vi "USBData_initialize.vi"(0 "USBData in":refnum<class "USBData.lvclass">, 2 "SeriesSetting":T2(array[cluster]) {"terminal type" items=["Default"=-1, "RSE"=10083, "NRSE"=10078, "Differential"=10106, "Pseudodifferential"=12529]}, 5 "BasePath":path, 7 "RunName":string, 9 "FileName":string, 11 "error in (no error)":errorcluster, 12 "RUN start time":timestamp) -> (3 "Status":T1(ring), 4 "USBData out":refnum<class "USBData.lvclass">, 6 "Labels(indicator)":string[](array[string]), 10 "LabelLD":string, 15 "error out":errorcluster)   [LabVIEW 2017, in "USBData.lvclass"]
uses:
  USBData.lvclass
  USBData.lvclass/USBData.ctl
panel:
  out "LeakDetetcorRead?":bool=TRUE
  out "FileFormatLD":string
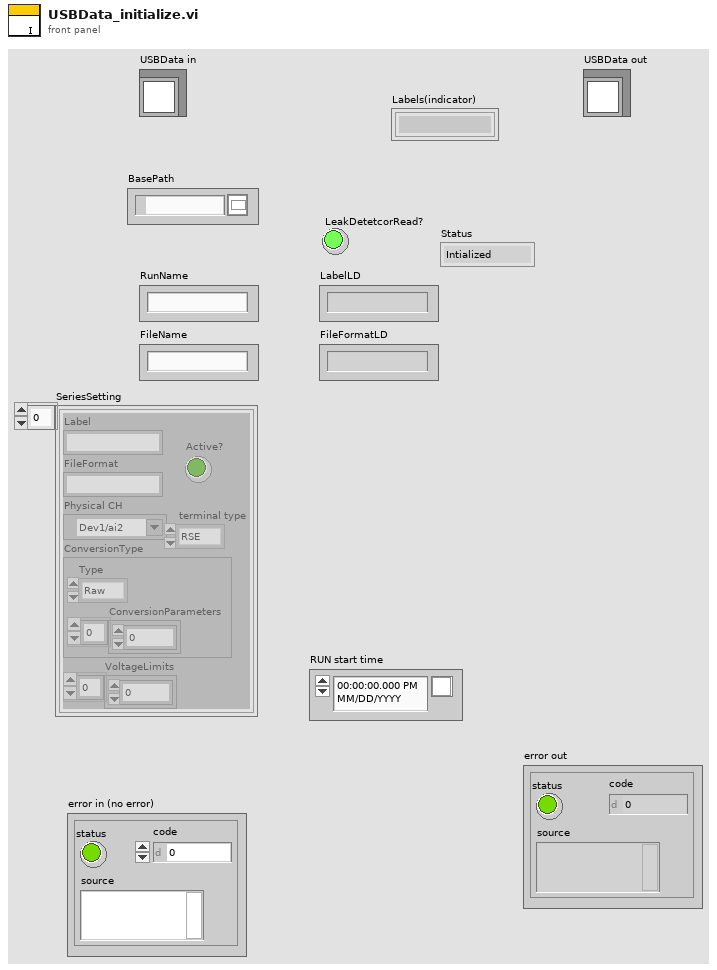
[diagram p1: front panel]
types:
  T1 = enum16{"Intialized", "Ready", "Measuring", "Terminated"}
  T2 = cluster{"Label":string, "FileFormat":string, "Active?":bool, "Physical CH":tag, " terminal type":i32, "ConversionType":cluster{"Type":enum16{"Raw", "SimpleProp", "CC-10_COMBINED", "CC-10_LOG", "LeakDet_EXP", "LeakDet_Mantissa", "Baratron"}, "ConversionParameters":dbl[]}, "VoltageLimits":dbl[]}[]
  T3 = enum16{"SimpleProp", "CC-10_COMBINED", "CC-10_LOG", "LeakDet_EXP", "LeakDet_Mantissa", "LeakDet_Full"}
  T4 = cluster{"Type":enum16{"Raw", "SimpleProp", "CC-10_COMBINED", "CC-10_LOG", "LeakDet_EXP", "LeakDet_Mantissa", "Baratron"}, "ConversionParameters":dbl[]}
  T5 = enum16{"Raw", "SimpleProp", "CC-10_COMBINED", "CC-10_LOG", "LeakDet_EXP", "LeakDet_Mantissa", "Baratron"}
  T6 = cluster{"Physical CH":tag, "Active?":bool, " terminal type":i32, "Type":enum16{"Raw", "SimpleProp", "CC-10_COMBINED", "CC-10_LOG", "LeakDet_EXP", "LeakDet_Mantissa", "Baratron"}, "ConversionParameters":dbl[]}[]
  T7 = enum16{"open", "replace", "create", "open or create", "replace or create", "replace or create with confirmation"}
  T8 = enum16{"Intialized", "Waiting", "Measuring", "Terminated"}
  T9 = cluster{"Physical CH":tag, "Active?":bool, " terminal type":i32, "Type":enum16{"Raw", "SimpleProp", "CC-10_COMBINED", "CC-10_LOG", "LeakDet_EXP", "LeakDet_Mantissa", "Baratron"}, "ConversionParameters":dbl[]}
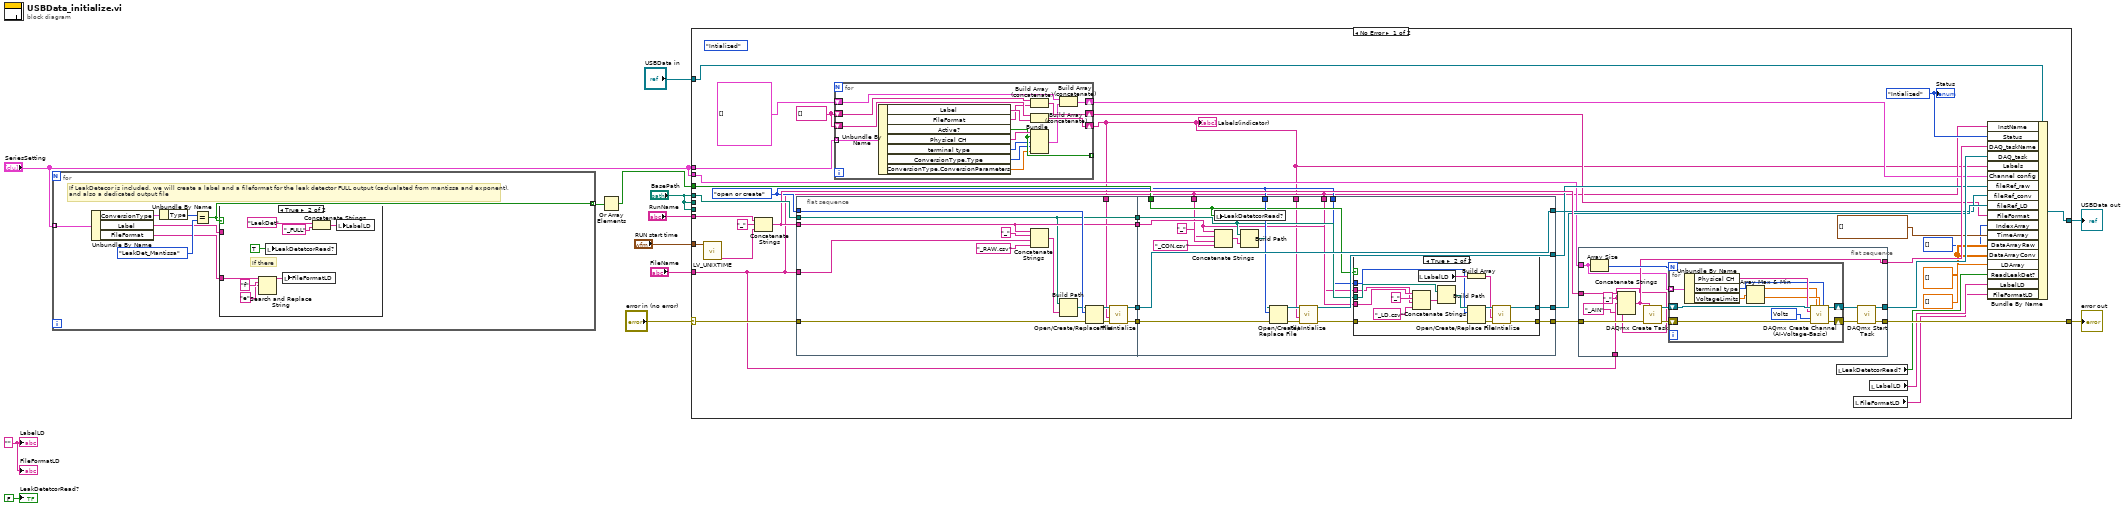
[diagram p0: block diagram]
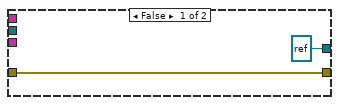
[diagram p3: hidden frame]
diagram:
  w6 = "" ("LabelLD")
  n1 = for {
    tunnel: "SeriesSetting" -> [w20] mode=indexing
    tunnel: [w14] -> w3 mode=indexing
    # "If LeakDetecor is included, we will create a label and a fileformat for the leak detector FULL output (caclualated from mantissa and exponent), \nand also a dedicated output file"
    n2 = Unbundle By Name(w20) -> ("ConversionType"=w19:T4, "Label"=w16:string, "FileFormat"=w15:string)
    n3 = Unbundle By Name(w19) -> ("Type"=w18:T5)
    n4 = Equal?(x=w18, y=T3."LeakDet_Mantissa") -> (x = y?=w14:bool)
    n5 = case shown="True" w14 {
      tunnel: w16 -> [_ _]
      tunnel: w15 -> [_ w22]
      frame False {
      }
      frame True {
        # "If there"
        n6 = Search and Replace String(input string=w22, search string="f", replace string="e" ("replace string (\"\")")) -> (result string=w25:string)  [unwired: 5 in, 3 out]
        n7 = local write "LeakDetetcorRead?"(TRUE ("LeakDetetcorRead?")) -> ()
        n8 = local write "FileFormatLD"(w25) -> ()
        n9 = Concatenate Strings("LaekDet" ("string"), "_FULL" ("string")) -> (w23:string)
        n10 = local write "LabelLD"(w23) -> ()
      }
    }
  }
  n11 = Or Array Elements(Boolean array=w3) -> (logical OR=w2:bool)
  n12 = case shown="No Error" "error in (no error)" {
    selector: "error in (no error)" -> [w60 w159]
    tunnel: [w62 w159] -> w12
    tunnel: "USBData in" -> [w53 w158]
    tunnel: [w43 w158] -> w10
    tunnel: "FileName" -> [w30 _]
    tunnel: "BasePath" -> [_ _]
    tunnel: "RunName" -> [w65 _]
    tunnel: "RUN start time" -> [w64 _]
    tunnel: "BasePath" -> [w61 _]
    tunnel: "BasePath" -> [_ _]
    tunnel: w2 -> [w39 _]
    tunnel: "SeriesSetting" -> [w37 _]
    tunnel: "SeriesSetting" -> [w36 _]
    frame No Error {
      w33 = T1."Intialized" ("Status")
      w35 = string[] [] ("Labels(indicator)")
      w38 = T7."open or create" ("operation (0:open)")
      w48 = dbl[][] [] ("DataArray")
      (unwired) T8."Intialized" ("Status")
      n13 = call "LV_UNIXTIME.vi"("current time"=w64) -> ("date/time string"=w66:string)  [unwired: 9 in, 1 out]
      n14 = Concatenate Strings(w65, "_" ("string"), w66) -> (w57:string)
      n15 = flat-sequence {
        tunnel: w57 -> [w87]
        tunnel: w61 -> [w86]
        tunnel: w60 -> [w94]
        tunnel: w38 -> [w93]
        tunnel: [w89] -> w59
        tunnel: [w88] -> w58
        tunnel: [w87] -> w56
        tunnel: [w86] -> w55
        tunnel: w30 -> [w84]
        tunnel: w29 -> [w82]
        tunnel: [w115] -> w44
        tunnel: w59 -> [w113]
        tunnel: w58 -> [w115]
        tunnel: w38 -> [w112]
        tunnel: [w108] -> w45
        tunnel: w56 -> [w106]
        tunnel: w55 -> [w107]
        tunnel: [w104] -> w54
        tunnel: [w103] -> w50
        tunnel: w39 -> [w102]
        tunnel: w38 -> [w101]
        tunnel: w30 -> [w98]
        tunnel: w30 -> [w99]
        tunnel: w29 -> [w96]
        frame #0 {
          n16 = Concatenate Strings(w87, "_" ("string"), w84, "_RAW.csv" ("string")) -> (w95:string)
          n17 = Build Path(base path=w86, name or relative path=w95) -> (appended path=w92:path)
          n18 = Open/Create/Replace File(file path (use dialog)=w92, error in=w94, operation (0:open)=w93) -> (refnum out=w90:refnum<file>, error out=w91:errorcluster)  [unwired: 3 in, 1 out]
          n19 = call "FileIntialize.vi"("Error In"=w91, "Labels"=w82, "refnum in"=w90) -> ("Error Out"=w89:errorcluster, "File Refnum"=w88:refnum<file>)  [unwired: 7 in]
        }
        frame #1 {
          n20 = local write "LeakDetetcorRead?"(w102) -> ()
          n21 = Concatenate Strings(w106, "_" ("string"), w98, "_CON.csv" ("string")) -> (w114:string)
          n22 = Build Path(base path=w107, name or relative path=w114) -> (appended path=w111:path)
          n23 = Open/Create/Replace File(file path (use dialog)=w111, error in=w113, operation (0:open)=w112) -> (refnum out=w109:refnum<file>, error out=w110:errorcluster)  [unwired: 3 in, 1 out]
          n24 = call "FileIntialize.vi"("Error In"=w110, "Labels"=w96, "refnum in"=w109) -> ("Error Out"=w105:errorcluster, "File Refnum"=w108:refnum<file>)  [unwired: 7 in]
          n25 = case shown="True" w102 {
            tunnel: w107 -> [_ w130]
            tunnel: w106 -> [_ w129]
            tunnel: w105 -> [w117 w124]
            tunnel: [w117 w123] -> w104
            tunnel: [refnum<file> refnum ("File Refnum") w122] -> w103
            tunnel: w101 -> [_ w121]
            tunnel: w99 -> [_ w118]
            frame False {
            }
            frame True {
              n26 = Concatenate Strings(w129, "_" ("string"), w118, "_LD.csv" ("string")) -> (w131:string)
              n27 = local read "LabelLD"() -> (w126:string)
              n28 = Build Path(base path=w130, name or relative path=w131) -> (appended path=w127:path)
              n29 = Build Array(w126) -> (w125:string[])
              n30 = Open/Create/Replace File(file path (use dialog)=w127, error in=w124, operation (0:open)=w121) -> (refnum out=w128:refnum<file>, error out=w132:errorcluster)  [unwired: 3 in, 1 out]
              n31 = call "FileIntialize.vi"("Error In"=w132, "Labels"=w125, "refnum in"=w128) -> ("Error Out"=w123:errorcluster, "File Refnum"=w122:refnum<file>)  [unwired: 7 in]
            }
          }
        }
      }
      n32 = for {
        tunnel: w36 -> [w81] mode=indexing
        shift-right: [w80] -> w29
        shift-left: w35 -> [w79]
        shift-right: [w75] -> w31
        shift-left: w35 -> [w76]
        tunnel: [w73] -> _ mode=indexing
        shift-right: [w71] -> w32
        shift-left: T6 [] -> [w70]
        n33 = Unbundle By Name(w81) -> ("Label"=w78:string, "FileFormat"=w77:string, "Active?"=w73:bool, "Physical CH"=w74:tag, "terminal type"=w72:i32, "ConversionType.Type"=w69:T5, "ConversionType.ConversionParameters"=w68:dbl[])
        n34 = Build Array (concatenate)(w76, w77) -> (w75:string[])
        n35 = Build Array (concatenate)(w79, w78) -> (w80:string[])
        n36 = Bundle("Physical CH"=w74, "Active?"=w73, "terminal type"=w72, "Type"=w69, "ConversionParameters"=w68) -> (w67:T9)  [unwired: 1 in]
        n37 = Build Array (concatenate)(w70, w67) -> (w71:T6)
      }
      "Labels(indicator)" <- w29
      n38 = flat-sequence {
        tunnel: w57 -> [w146]
        tunnel: [w140] -> w62
        tunnel: [w139] -> w52
        tunnel: [w138] -> w51
        tunnel: w54 -> [w137]
        tunnel: w37 -> [w136]
        tunnel: w30 -> [w135]
        frame #0 {
          w134 = "_" ("string")
          n39 = Array Size(array=w136) -> (size(s)=w145:i32)
          n40 = Concatenate Strings(w146, w134, w135, w134, "_AIN" ("new task name")) -> (w139:string)
          n41 = call <vilib>:"DAQmx Create Task.vi"("new task name"=w139, "error in"=w137) -> ("task out"=w144:refnum<k21>, "error out"=w143:errorcluster)  [unwired: 12 in]
          n42 = for {
            N: w145 -> [_]
            shift-right: [w155] -> w142
            shift-left: w144 -> [w156]
            shift-right: [w153] -> w141
            shift-left: w143 -> [w154]
            tunnel: w136 -> [w152] mode=indexing
            w157 = 10348 items=["Volts"=10348, "From Custom Scale"=10065] ("units")
            n43 = Unbundle By Name(w152) -> ("Physical CH"=w151:tag, "terminal type"=w150:i32, "VoltageLimits"=w149:dbl[])
            n44 = Array Max & Min(array=w149) -> (max value=w147:dbl, min value=w148:dbl)  [unwired: 2 out]
            n45 = call <vilib>:"DAQmx Create Channel (AI-Voltage-Basic).vi"("task in"=w156, "maximum value"=w147, "minimum value"=w148, "input terminal configuration"=w150, "physical channels"=w151, "units"=w157, "error in"=w154) -> ("task out"=w155:refnum<k21>, "error out"=w153:errorcluster)  [unwired: 7 in]
          }
          n46 = call <vilib>:"DAQmx Start Task.vi"("task/channels in"=w142, "error in"=w141) -> ("task out"=w138:refnum<k21>, "error out"=w140:errorcluster)  [unwired: 12 in]
        }
      }
      n47 = local read "LeakDetetcorRead?"() -> (w42:bool)
      n48 = local read "FileFormatLD"() -> (w40:string)
      n49 = local read "LabelLD"() -> (w41:string)
      n50 = Bundle By Name(cluster=w53, "InstName"=w30, "Status"=w33, "DAQ_taskName"=w52, "DAQ_task"=w51, "Labels"=w29, "Channel config"=w32, "fileRef_raw"=w44, "fileRef_conv"=w45, "fileRef_LD"=w50, "FileFormat"=w31, "IndexArray"=i64[] [], "TimeArray"=timestamp[] [], "DataArrayRaw"=w48, "DataArrayConv"=w48, "LDArray"=dbl[] [], "ReadLeakDet?"=w42, "LabelLD"=w41, "FileFormatLD"=w40) -> (w43:refnum<class "USBData.lvclass">)
      "Status" <- w33
    }
    frame Error {
    }
  }
  "error out" <- w12
  "USBData out" <- w10
  "FileFormatLD" <- w6
  "LabelLD" <- w6
  "LeakDetetcorRead?" <- FALSE ("LeakDetetcorRead?")
